vi "Set niRfsgBT Handle.vi"(8 "error in (no error)":errorcluster, 10 "InstDriver Handle in":T1, 11 "niDTS BT INSTR RX in":refnum<class "niDTS BT INSTR RX.lvclass">) -> (0 "error out":errorcluster, 3 "niDTS BT INSTR RX out":refnum<class "niDTS BT INSTR RX.lvclass">)   [LabVIEW 2015, in "niDTS BT.lvlib" / "niDTS BT INSTR RX.lvclass"]
uses:
  niDTS BT INSTR RX.lvclass
  RiviInstDriver/niRfsgBT/Includes/niRfsgBt INC Handle.ctl
  RiviInstDriver/niRfsgBT/Objects/niRfsgBt.lvclass
  niDTS BT INSTR RX.lvclass/niDTS BT INSTR RX.ctl
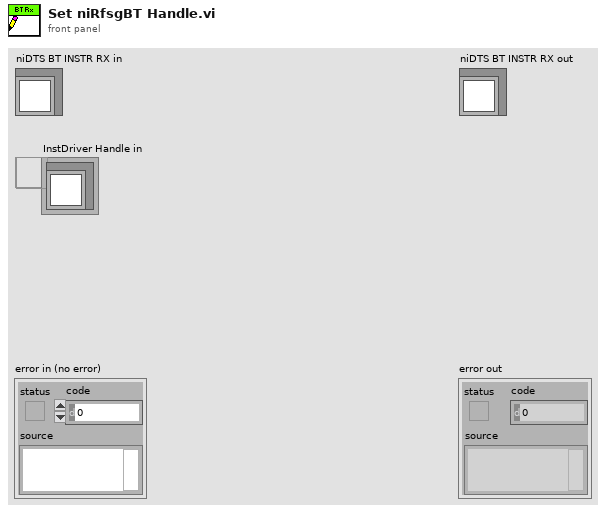
[diagram p1: front panel]
types:
  T1 = typedef "niRfsgBT.lvclass/niRfsgBT INC Handle.ctl" = refnum<data-value>
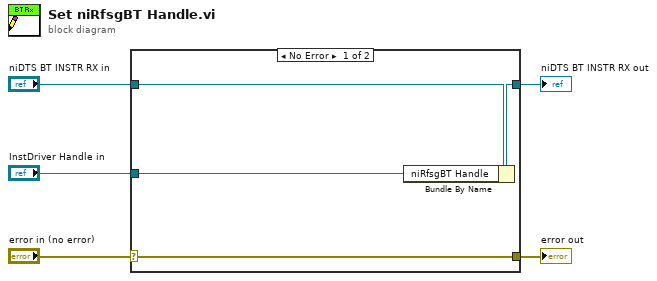
[diagram p0: block diagram]
diagram:
  n1 = case shown="No Error" "error in (no error)" {
    selector: "error in (no error)" -> [w9 w10]
    tunnel: [w9 w10] -> w4
    tunnel: [w7 w11] -> w2
    tunnel: "niDTS BT INSTR RX in" -> [w8 w11]
    tunnel: "InstDriver Handle in" -> [w6 _]
    frame No Error {
      n2 = Bundle By Name(cluster=w8, "niRfsgBT Handle"=w6) -> (w7:refnum<class "niDTS BT INSTR RX.lvclass">)
    }
    frame Error {
    }
  }
  "error out" <- w4
  "niDTS BT INSTR RX out" <- w2
